vi "Intake.vi"(8 "Intake Out Full":bool, 9 "Intake Out 1/4":bool, 10 "Intake In Full":bool, 11 "Intake In 1/4":bool) -> ()   [LabVIEW 2017]
uses:
  Robot Global Data.vi
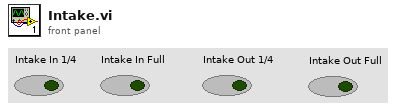
[diagram p1: front panel]
types:
  T1 = typedef "WPI_MotorControlDeviceRef.ctl" = cluster{"DeviceStatus":errorcluster, "Type":T2, "PWM":cluster{"PWM Channel":T3, "DeadBand":T4}, "CAN":cluster{"Device Number":u8, "SetOutput VI Ref":variant, "GetOutput VI Ref":variant, "Enable VI Ref":variant, "Disable VI Ref":variant, "Data":variant}, "Invert":bool, "DIO PWM":cluster{"PWM \"Enable\" Channel":T3, "DIOChannel":T5, "PWM Rate":dbl}}
  T2 = typedef "WPI_MotorControlType.ctl" = enum16{"PWM", "CAN", "DIO PWM"}
  T3 = typedef "FPGA_DIOPWMChannel.ctl" = enum8{"PWM 0", "PWM 1", "PWM 2", "PWM 3", "PWM 4", "PWM 5", "PWM 6", "PWM 7", "PWM 8", "PWM 9", "PWM MXP 0", "PWM MXP 1", "PWM MXP 2", "PWM MXP 3", "PWM MXP 4", "PWM MXP 5", "PWM MXP 6", "PWM MXP 7", "PWM MXP 8", "PWM MXP 9", "Invalid"}
  T4 = typedef "WPI_PWMDeadband.ctl" = cluster{"Name":string, "maxPositivePwm":i32, "minPositivePwm":i32, "centerPwm":i32, "maxNegativePwm":i32, "minNegativePwm":i32, "angularRange":u16}
  T5 = typedef "FPGA_DIOChannel.ctl" = enum8{"DIO 0", "DIO 1", "DIO 2", "DIO 3", "DIO 4", "DIO 5", "DIO 6", "DIO 7", "DIO 8", "DIO 9", "DIO MXP 0", "DIO MXP 1", "DIO MXP 2", "DIO MXP 3", "DIO MXP 4", "DIO MXP 5", "DIO MXP 6", "DIO MXP 7", "DIO MXP 8", "DIO MXP 9", "DIO MXP 10", "DIO MXP 11", "DIO MXP 12", "DIO MXP 13", "DIO MXP 14", "DIO MXP 15", "SPI Port CS1", "SPI Port CS2", "SPI Port CS3", "SPI Port MISO", "SPI Port MOSI", "Invalid"}
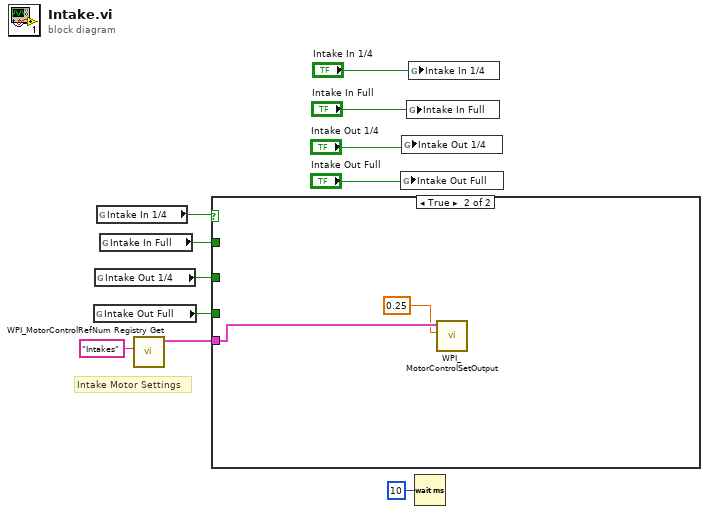
[diagram p0: block diagram]
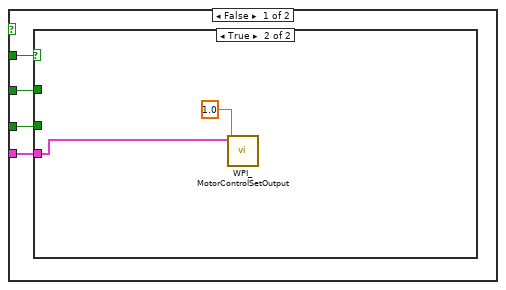
[diagram p2: hidden frame]
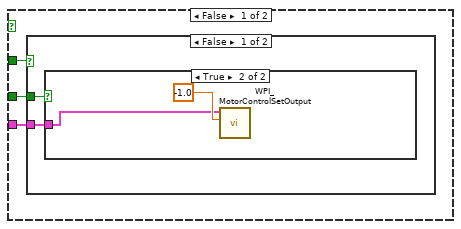
[diagram p3: hidden frame]
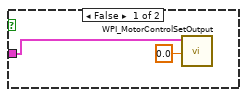
[diagram p4: hidden frame]
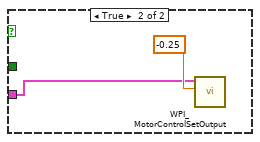
[diagram p5: hidden frame]
diagram:
  # "Intake Motor Settings"
  n1 = global read "Robot Global Data.vi" "Intake Out Full"() -> (w11:bool)
  n2 = global read "Robot Global Data.vi" "Intake Out 1/4"() -> (w10:bool)
  n3 = global read "Robot Global Data.vi" "Intake In 1/4"() -> (w1:bool)
  n4 = global read "Robot Global Data.vi" "Intake In Full"() -> (w9:bool)
  n5 = call <vilib>:"WPI_MotorControlRefNum Registry Get.vi"("refnum name"="Intakes") -> ("MotorControlDevRef"=w7:T1)  [unwired: 9 in, 1 out]
  n6 = case shown="True" w1 {
    tunnel: w11 -> [w15 _]
    tunnel: w10 -> [w14 _]
    tunnel: w9 -> [w13 _]
    tunnel: w7 -> [w12 w30]
    frame False {
      n7 = case shown="True" w13 {
        tunnel: w15 -> [w18 _]
        tunnel: w14 -> [w17 _]
        tunnel: w12 -> [w16 w27]
        frame False {
          n8 = case shown="False" w17 {
            tunnel: w18 -> [w20 _]
            tunnel: w16 -> [w19 w25]
            frame False {
              n9 = case shown="True" w20 {
                tunnel: w19 -> [w21 w23]
                frame False {
                  n10 = call <vilib>:"WPI_MotorControlSetOutput.vi"("Output"=0.0, "MotorControlDevRef"=w21) -> ()  [unwired: 7 in, 3 out]
                }
                frame True {
                  n11 = call <vilib>:"WPI_MotorControlSetOutput.vi"("Output"=-1.0, "MotorControlDevRef"=w23) -> ()  [unwired: 7 in, 3 out]
                }
              }
            }
            frame True {
              n12 = call <vilib>:"WPI_MotorControlSetOutput.vi"("Output"=-0.25, "MotorControlDevRef"=w25) -> ()  [unwired: 7 in, 3 out]
            }
          }
        }
        frame True {
          n13 = call <vilib>:"WPI_MotorControlSetOutput.vi"("Output"=1.0, "MotorControlDevRef"=w27) -> ()  [unwired: 7 in, 3 out]
        }
      }
    }
    frame True {
      n14 = call <vilib>:"WPI_MotorControlSetOutput.vi"("Output"=0.25, "MotorControlDevRef"=w30) -> ()  [unwired: 7 in, 3 out]
    }
  }
  n15 = global write "Robot Global Data.vi" "Intake Out Full"("Intake Out Full") -> ()
  n16 = global write "Robot Global Data.vi" "Intake Out 1/4"("Intake Out 1/4") -> ()
  n17 = global write "Robot Global Data.vi" "Intake In Full"("Intake In Full") -> ()
  n18 = global write "Robot Global Data.vi" "Intake In 1/4"("Intake In 1/4") -> ()
  n19 = Wait (ms)(milliseconds to wait=u32 10) -> ()  [unwired: 1 out]
